vi "Read Upper Limit.vi"(8 "error in (no error)":errorcluster, 11 "Test Numeric in":refnum<class "Test Numeric.lvclass">) -> (0 "error out":errorcluster, 2 "Abs_Numeric.lvclass":refnum<class "Abs_Numeric.lvclass">, 3 "Test Numeric out":refnum<class "Test Numeric.lvclass">)   [LabVIEW 2021, in "BT.lvlib" / "Test Numeric.lvclass"]
uses:
  Test Numeric.lvclass
  LV_Abstract/Source/Abs_Types/Numeric/Abs_Numeric.lvclass
  Test Numeric.lvclass/Test Numeric.ctl
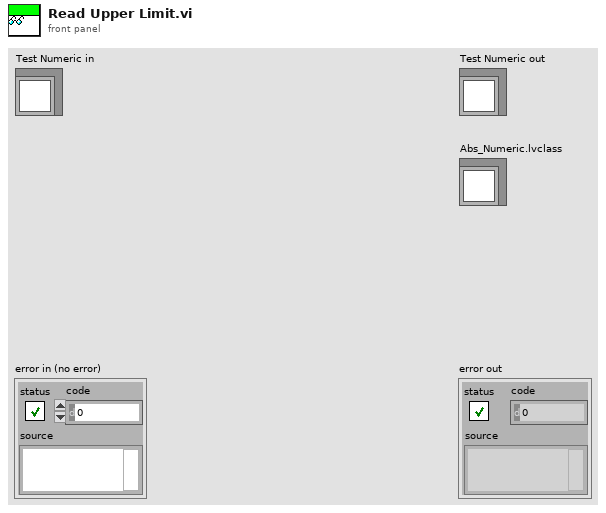
[diagram p1: front panel]
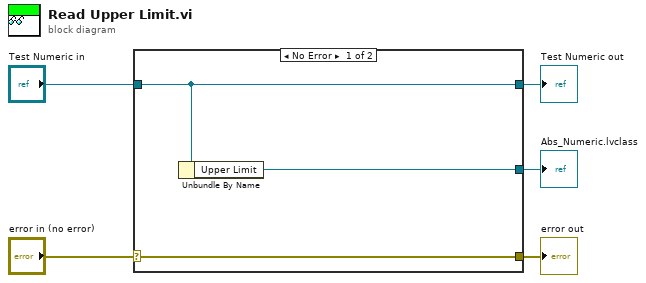
[diagram p0: block diagram]
diagram:
  n1 = case shown="No Error" "error in (no error)" {
    selector: "error in (no error)" -> [w8 w9]
    tunnel: [w8 w9] -> w4
    tunnel: [w7 w10] -> w2
    tunnel: "Test Numeric in" -> [w7 w10]
    tunnel: [w6 _] -> w1
    frame No Error {
      n2 = Unbundle By Name(w7) -> ("Upper Limit"=w6:refnum<class "Abs_Numeric.lvclass">)
    }
    frame Error {
    }
  }
  "error out" <- w4
  "Test Numeric out" <- w2
  "Abs_Numeric.lvclass" <- w1
